vi "Get Debug Log.vi"(8 "error in (no error)":errorcluster, 10 "Node":string, 11 "System Status Module in":refnum<class "System Status Module.lvclass">) -> (0 "error out":errorcluster, 3 "System Status Module out":refnum<class "System Status Module.lvclass">)   [LabVIEW 2020, in "VolatusGUI.lvlib" / "System Status Module.lvclass"]
uses:
  System Status Module.lvclass
  C:/dev/lv20CE/relink/lv-volatus/Volatus/Module/Module.lvclass
  lv-cdm/CDM-Config/ISO8601 Config.ctl
  lv-cdm/CDM-Config/Format.ctl
  lv-cdm/CDM-Config/Precision.ctl
  lv-cdm/CDM-Config/Timezone.ctl
  Volatus/Module/Module.lvclass/Module.ctl
  Volatus/VolatusAPI/VolatusAPI.lvclass/VolatusAPI.ctl
  lv-cdm/CDM-Config/ISO-8601 Format Strings.vi
  System Status Module.lvclass/System Status Module.ctl
  Volatus/Module/Module.lvclass
  Volatus/VolatusAPI/VolatusAPI.lvclass
  <vilib>/httpClient/LabVIEWHTTPClient.lvlib
  VolatusConfig/Node/Node Config.lvclass
  lv-cdm/CDM-Config/CDM-Config.lvlib
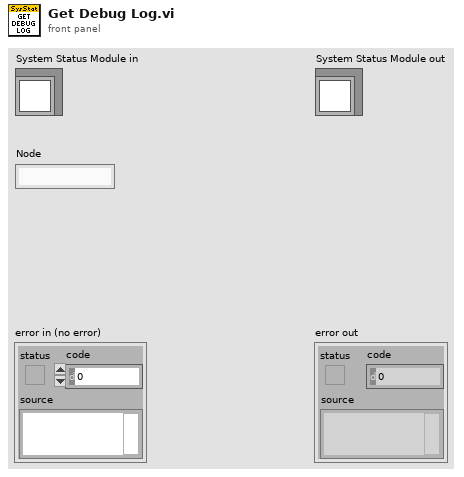
[diagram p1: front panel]
types:
  T1 = typedef "CDM-Config.lvlib/ISO8601 Config.ctl" = cluster{"Format":T2, "Precision":T3, "Timezone":T4}
  T2 = typedef "CDM-Config.lvlib/Format.ctl" = enum16{"Extended", "Basic"}
  T3 = typedef "CDM-Config.lvlib/Precision.ctl" = enum16{"Millisecond", "Second", "Minute", "Hour", "Day"}
  T4 = typedef "CDM-Config.lvlib/Timezone.ctl" = enum16{"UTC", "Local"}
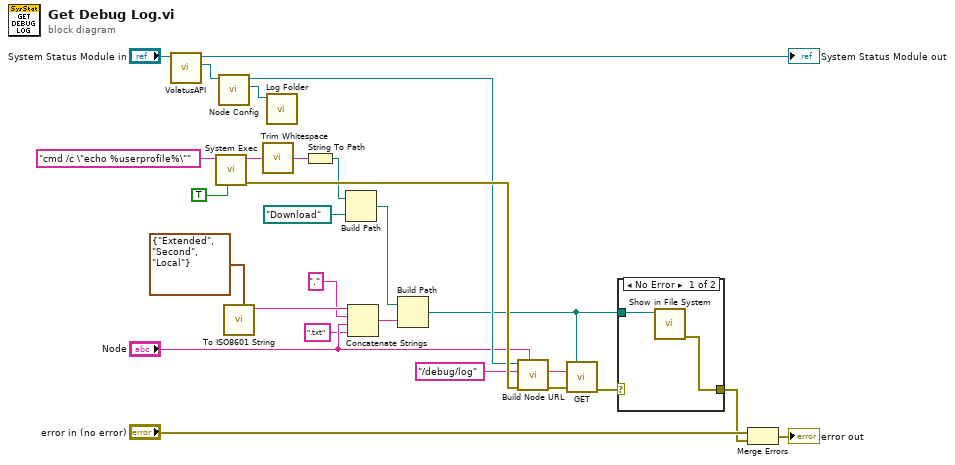
[diagram p0: block diagram]
diagram:
  n1 = call "VolatusAPI.vi"("Module in"="System Status Module in") -> ("VolatusAPI"=w21:refnum<class "VolatusAPI.lvclass">, "Module out"=→"System Status Module out":refnum<class "System Status Module.lvclass">)  [unwired: 9 in]
  n2 = call <vilib>:"System Exec.vi"("run minimized? (F)"=TRUE, "command line"="cmd /c \"echo %userprofile%\"") -> ("error out"=w27:errorcluster, "standard output"=w16:string)  [unwired: 6 in, 2 out]
  n3 = call "Node Config.vi"("VolatusAPI in"=w21) -> ("Node Config"=w19:refnum<class "Node Config.lvclass">, "VolatusAPI out"=w20:refnum<class "VolatusAPI.lvclass">)  [unwired: 9 in]
  n4 = call "To ISO8601 String.vi"("Format Config"=T1 {"Format"=enum."Extended", "Precision"=enum."Second", "Timezone"=enum."Local"}) -> ("ISO 8601"=w12:string)  [unwired: 10 in]
  n5 = call <vilib>:"Trim Whitespace.vi"("string"=w16) -> ("trimmed string"=w1:string)  [unwired: 1 in]
  n6 = call "Log Folder.vi"("Node Config in"=w19) -> ()  [unwired: 8 in, 3 out]
  n7 = String To Path(string=w1) -> (path=w15:path)
  n8 = Build Path(base path=w15, name or relative path=path "Download") -> (appended path=w8:path)
  n9 = Concatenate Strings(w12, "." ("string"), "Node", ".txt" ("string")) -> (w7:string)
  n10 = Build Path(base path=w8, name or relative path=w7) -> (appended path=w4:path)
  n11 = call "Build Node URL.vi"("Node Name"="Node", "error in (no error)"=w27, "Path"="/debug/log", "VolatusAPI in"=w20) -> ("error out"=w6:errorcluster, "Request URL"=w22:string)  [unwired: 5 in, 1 out]
  n12 = call <vilib>:"GET.vi"("output file"=w4, "url"=w22, "error in (no error)"=w6) -> ("error out"=w5:errorcluster)  [unwired: 9 in, 3 out]
  n13 = case shown="No Error" w5 {
    selector: w5 -> [_ w30]
    tunnel: w4 -> [w29 _]
    tunnel: [w28 w30] -> w2
    frame No Error {
      n14 = call <vilib>:"Show in File System.vi"("file or directory path"=w29) -> ("error out"=w28:errorcluster)  [unwired: 10 in]
    }
    frame Error {
    }
  }
  n15 = Merge Errors("error in (no error)", w2) -> (→"error out":errorcluster)
